vi "Save_RegDests.vi"(8 "error in (no error)":errorcluster, 11 "Class in":refnum<class "IB_MSI.lvclass">) -> (0 "error out":errorcluster, 3 "Class out":refnum<class "IB_MSI.lvclass">)   [LabVIEW 2020, in "IB_MSI.lvclass"]
uses:
  <vilib>/AppBuilder/IB_Classes/MSI/IB_MSI.lvclass
  <vilib>/AppBuilder/IB_Classes/MSI/IB_MSI.lvclass/IB_MSI.ctl
  <vilib>/AppBuilder/IB_Classes/Installer/Installer.lvclass
  <vilib>/AppBuilder/IB_Classes/RegDest/IB_RegDest.lvclass
  e:/builds/penguin/labview/branches/2020/dev/dist/vi.lib/AppBuilder/IB_Classes/Installer/Installer.lvclass
  e:/builds/penguin/labview/branches/2020/dev/dist/vi.lib/AppBuilder/IB_Classes/MSI/IB_MSI.lvclass
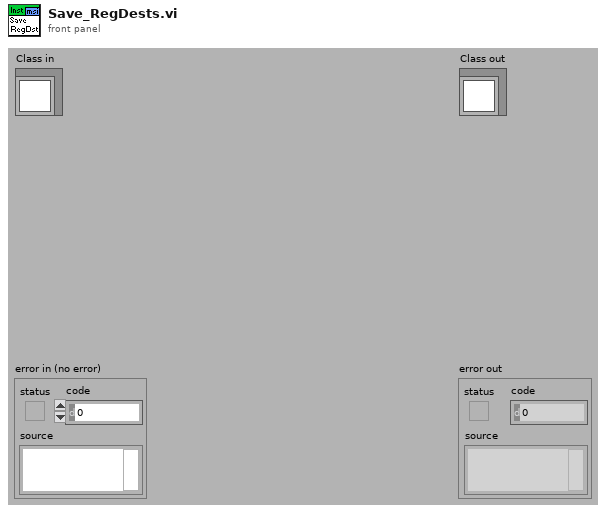
[diagram p1: front panel]
types:
  T1 = typedef "IB_Installer.ctl" = cluster{"Destination":refnum<class "IB_Destination.lvclass">[], "Source":refnum<class "IB_Source.lvclass">[], "buildObject":T2, "defaultDir":string, "platform":string, "author":string, "productName":string, "buildSpecName":string, "hide":bool, "requireLVDevSys":bool, "autoIncrement":bool, "includeError":bool, "readmeID":string, "buildLocation":path, "readmePath":path, "mediaSize":u16, "language":T3, "productVersion":T4, "preview":bool, "programmatic":bool, "progressBarEvents":T5, "userLog_Path":path, "shortcutAddresses":T7[], "EXE_Install Address":string, "EXE_Uninstall Address":string, "additional NIPaths":refnum<class "Dest_NI_NIPath.lvclass">[], "web service itemIDs":string[], "installerName":string}
  T2 = typedef "ItemRef.ctl" = u64
  T3 = typedef "CDK_sTypeDef_Languages.ctl" = u16
  T4 = typedef "CDK_sTypeDef_ProductVersion.ctl" = cluster{"Major":u8, "Minor":u8, "Update":u16}
  T5 = typedef "provcom_ProgressBar_Events.ctl" = cluster{"newJob":refnum<user-event>, "newItem":refnum<user-event>, "errorMsg":T6, "cancel":refnum<user-event>}
  T6 = typedef "mxLvBuildError.ctl" = refnum<user-event>
  T7 = typedef "CDK_sTypeDef_ShortcutAddress.ctl" = cluster{"file":string, "shortcut":string}
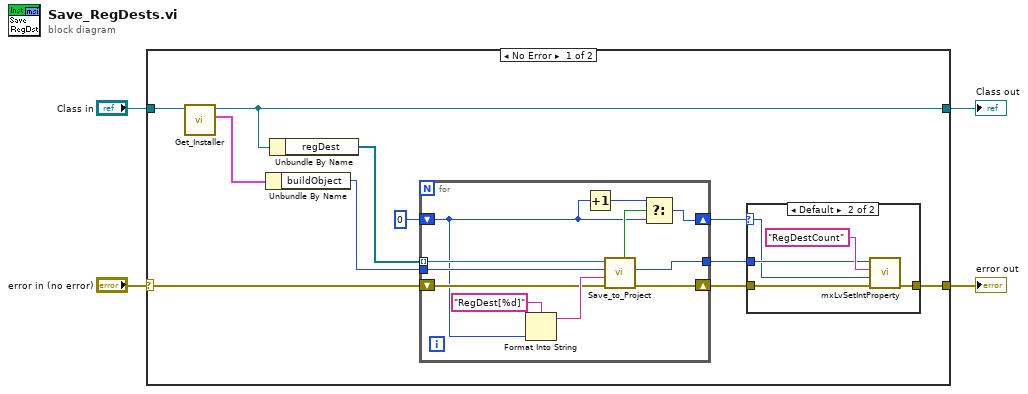
[diagram p0: block diagram]
diagram:
  n1 = case shown="No Error" "error in (no error)" {
    selector: "error in (no error)" -> [w5 w34]
    tunnel: [w7 w34] -> w3
    tunnel: [w14 w33] -> w1
    tunnel: "Class in" -> [w12 w33]
    frame No Error {
      n2 = call <vilib>:"Get_Installer.vi"("Installer in"=w12) -> ("data"=w13:T1, "Installer out"=w14:refnum<class "IB_MSI.lvclass">)  [unwired: 8 in, 1 out]
      n3 = Unbundle By Name(w13) -> ("buildObject"=w11:T2)
      n4 = Unbundle By Name(w14) -> ("regDest"=w15:refnum<class "IB_RegDest.lvclass">[])
      n5 = for {
        tunnel: w15 -> [w30] mode=indexing
        tunnel: w11 -> [w29]
        shift-right: [w32] -> w8
        shift-left: w5 -> [w27]
        shift-right: [w24] -> w6
        shift-left: 0 -> [w22]
        tunnel: [w23] -> w9
        n6 = Format Into String(format string="RegDest[%d]", w22) -> (resulting string=w28:string)  [unwired: 2 in, 1 out]
        n7 = Increment(x=w22) -> (x+1=w25:i32)
        n8 = call-dynamic "Save_to_Project.vi"("error in (no error)"=w27, "index in"=w28, "buildObject"=w29, "IB_RegDest in"=w30) -> ("error out"=w32:errorcluster, "buildObject out"=w23:T2, "saved?"=w26:bool)  [unwired: 3 in, 2 out]
        n9 = Select(t=w25, s=w26, f=w22) -> (s? t:f=w24:i32)
      }
      n10 = case shown="Default" w6 {
        selector: w6 -> [_ w17]
        tunnel: w9 -> [_ w20]
        tunnel: w8 -> [w16 w19]
        tunnel: [w16 w18] -> w7
        frame 0 {
        }
        frame Default {
          n11 = call <resource>:"mxLvSetIntProperty.vi"("error in"=w19, "Value (0)"=w17, "Tag"="RegDestCount", "Item"=w20) -> ("error out"=w18:errorcluster)  [unwired: 1 in, 6 out]
        }
      }
    }
    frame Error {
    }
  }
  "error out" <- w3
  "Class out" <- w1
